vi "Close Hardware.vi"(8 "error in (no error)":errorcluster, 11 "Inst.Krohn-Hite-7008 in":refnum<class "Inst.Krohn-Hite-7008.lvclass">) -> (0 "error out":errorcluster, 3 "Inst.Krohn-Hite-7008 out":refnum<class "Inst.Krohn-Hite-7008.lvclass">)   [LabVIEW 2019, in "Inst.Krohn-Hite-7008.lvclass"]
uses:
  Inst.Krohn-Hite-7008.lvclass
  Inst.Krohn-Hite-7008.lvclass/Inst.Krohn-Hite-7008.ctl
  <userlib>/LevyLab/Instrument Framework/Instrument Types/VSource/Instrument.VSource.lvclass
  KH7008/KH7008.lvlib
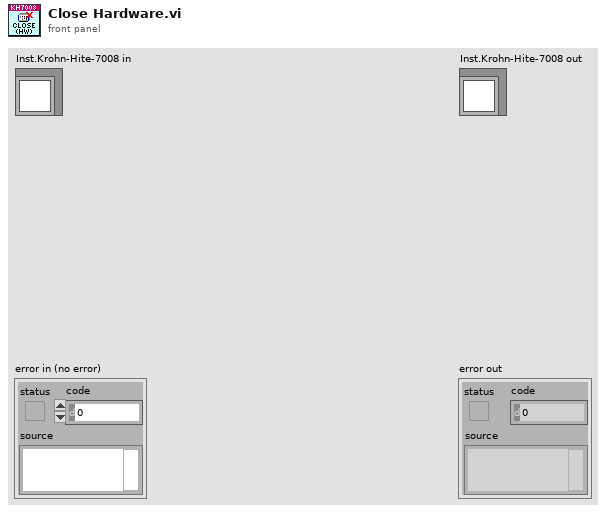
[diagram p1: front panel]
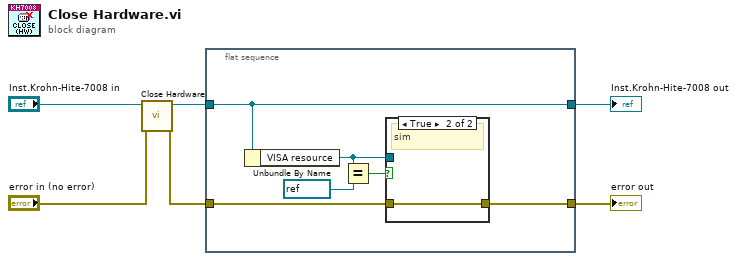
[diagram p0: block diagram]
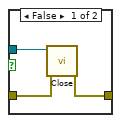
[diagram p2: hidden frame]
diagram:
  n1 = call-parent "Close Hardware.vi"("error in (no error)"="error in (no error)", "Instrument in"="Inst.Krohn-Hite-7008 in") -> ("error out"=w4:errorcluster, "Instrument out"=w2:refnum<class "Inst.Krohn-Hite-7008.lvclass">)  [unwired: 8 in]
  n2 = flat-sequence {
    tunnel: w4 -> [w11]
    tunnel: [w10] -> w3
    tunnel: w2 -> [w12]
    tunnel: [w12] -> w1
    frame #0 {
      n3 = Unbundle By Name(w12) -> ("VISA resource"=w9:refnum<visa-resource-name>)
      n4 = Equal?(x=w9, y=refnum<visa-resource-name> "sim" ("VISA resource name out")) -> (x = y?=w7:bool)
      n5 = case shown="True" w7 {
        tunnel: w11 -> [w15 w16]
        tunnel: [w14 w16] -> w10
        tunnel: w9 -> [w13 _]
        frame False {
          n6 = call "Close.vi"("error in (no error)"=w15, "VISA resource name"=w13) -> ("error out"=w14:errorcluster)  [unwired: 9 in]
        }
        frame True {
          # "sim"
        }
      }
    }
  }
  "error out" <- w3
  "Inst.Krohn-Hite-7008 out" <- w1
